vi "HEWH Assemble HEWH Diagnostics Data.vi"(8 "Error In":errorcluster, 11 "Water Heater GEA2 Data in":T1 {"Hyperterminal Data"."CRC" format="%x"; "Hyperterminal Data"."Length" format="%x"; "Hyperterminal Data"."Command" format="%x"; "Hyperterminal Data"."Destination" format="%x"; "Hyperterminal Data"."Source" format="%x"}) -> (0 "Error Out":errorcluster, 3 "Hyperterminal Data":string[][](array[string]))   [LabVIEW 2018]
uses:
  Utility/GEA2 Commands/HEWH/Type Definitions/GEA2 Commands WaterHeater GEA2 Data.ctl
  Utility/GEA2 Commands/HEWH/Type Definitions/GEA2 Commands Button Status.ctl
  Utility/GEA2 Commands/HEWH/Type Definitions/GEA2 Commands Status Query.ctl
  Utility/GEA2 Commands/HEWH/Type Definitions/GEA2 Commands Service Error Codes.ctl
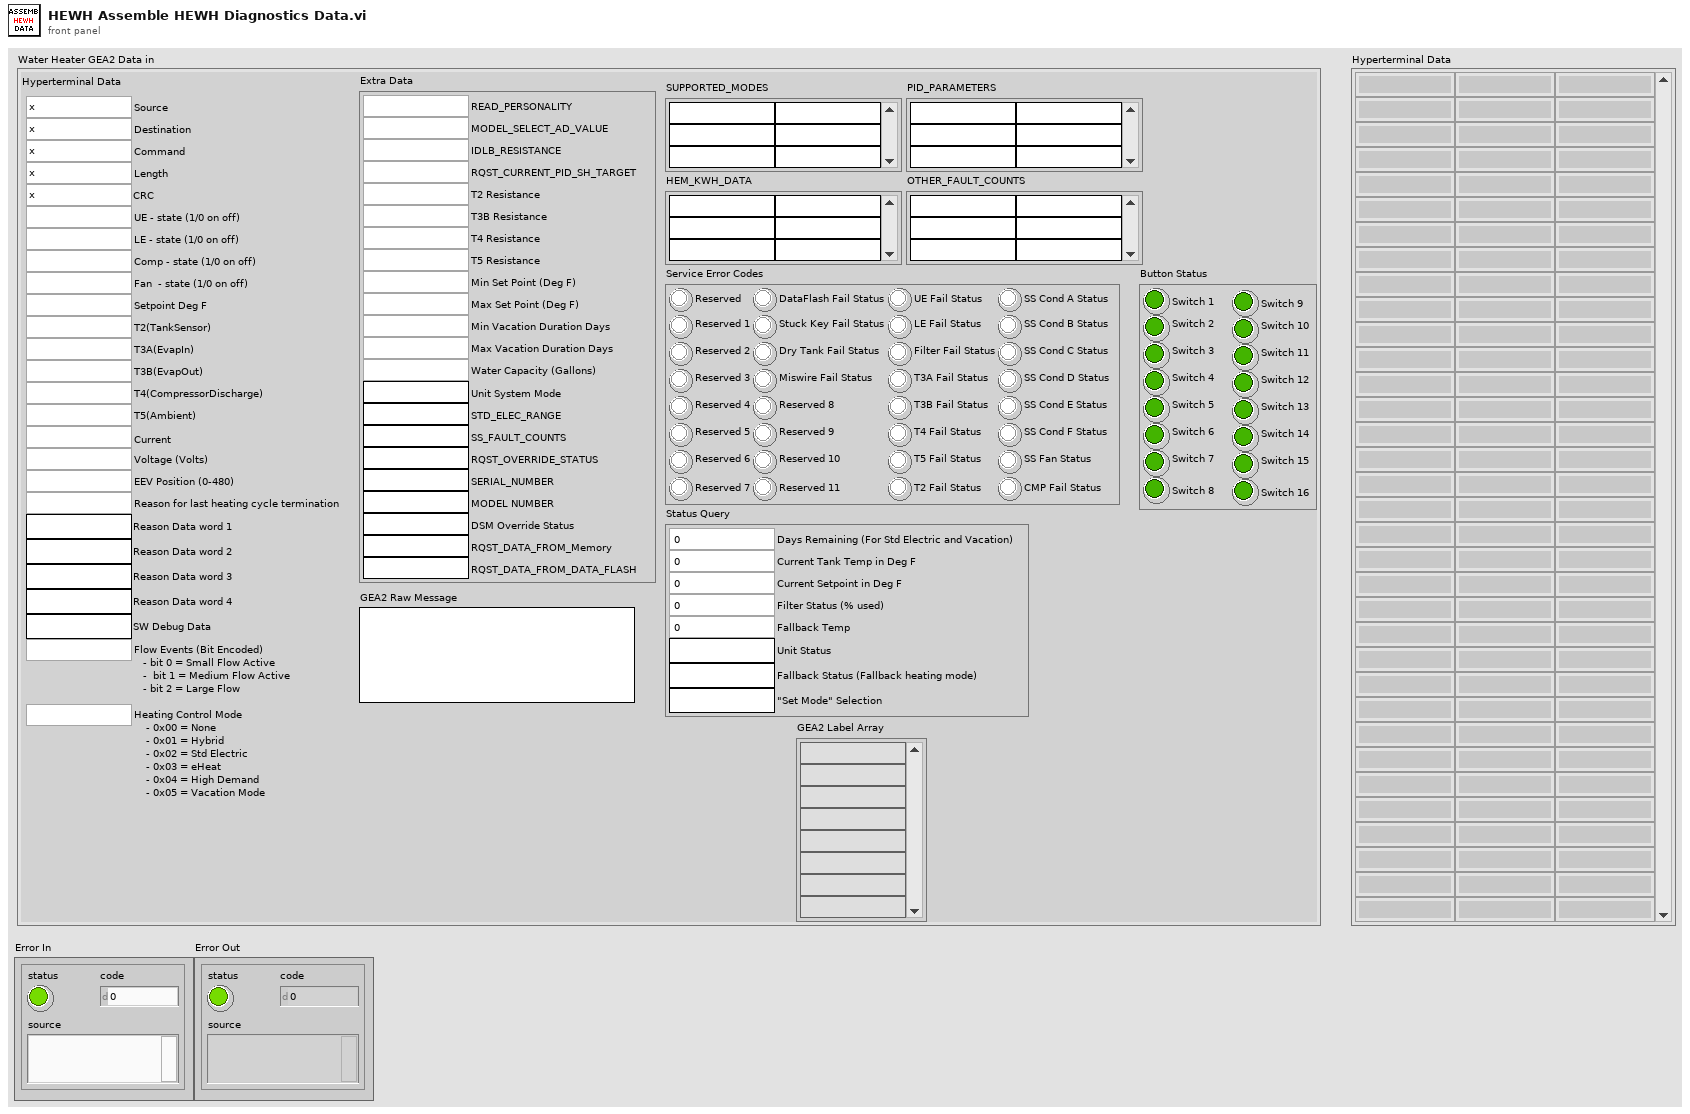
[diagram p1: front panel]
types:
  T1 = typedef "GEA2 Commands WaterHeater GEA2 Data.ctl" = cluster{"GEA2 Label Array":string[], "PID_PARAMETERS":string[][], "SUPPORTED_MODES":string[][], "Button Status":T2, "Status Query":T3, "Service Error Codes":T4, "HEM_KWH_DATA":string[][], "OTHER_FAULT_COUNTS":string[][], "GEA2 Raw Message":string, "Hyperterminal Data":cluster{"Source":u8, "Destination":u8, "Command":u8, "Length":u8, "CRC":u16, "UE - state (1/0 on off)":u8, "LE - state (1/0 on off)":u8, "Comp - state (1/0 on off)":u8, "Fan  - state (1/0 on off)":u8, "Setpoint Deg F":i32, "T2(TankSensor)":dbl, "T3A(EvapIn)":dbl, "T3B(EvapOut)":dbl, "T4(CompressorDischarge)":dbl, "T5(Ambient)":dbl, "Current":dbl, "Voltage (Volts)":u16, "EEV Position (0-480)":u16, "Reason for last heating cycle termination":u16, "Reason Data word 1":string, "Reason Data word 2":string, "Reason Data word 3":string, "Reason Data word 4":string, "SW Debug Data":string, "Flow Events (Bit Encoded)":u16, "Heating Control Mode":u16}, "Extra Data":cluster{"Water Capacity (Gallons)":u32, "Max Vacation Duration Days":u32, "Min Vacation Duration Days":u32, "Max Set Point (Deg F)":u32, "Min Set Point (Deg F)":u32, "T5 Resistance":u32, "T4 Resistance":u32, "T3B Resistance":u32, "T2 Resistance":u32, "STD_ELEC_RANGE":string, "SS_FAULT_COUNTS":string, "SERIAL_NUMBER":string, "READ_PERSONALITY":u8, "RQST_OVERRIDE_STATUS":string, "MODEL_SELECT_AD_VALUE":u32, "MODEL NUMBER":string, "IDLB_RESISTANCE":u32, "DSM Override Status":string, "RQST_DATA_FROM_Memory":string, "RQST_DATA_FROM_DATA_FLASH":string, "RQST_CURRENT_PID_SH_TARGET":u16, "Unit System Mode":string}}
  T2 = typedef "GEA2 Commands Button Status.ctl" = cluster{"Switch 1":bool, "Switch 2":bool, "Switch 3":bool, "Switch 4":bool, "Switch 5":bool, "Switch 6":bool, "Switch 7":bool, "Switch 8":bool, "Switch 9":bool, "Switch 10":bool, "Switch 11":bool, "Switch 12":bool, "Switch 13":bool, "Switch 14":bool, "Switch 15":bool, "Switch 16":bool}
  T3 = typedef "GEA2 Commands Status Query.ctl" = cluster{"Days Remaining (For Std Electric and Vacation)":u8, "Unit Status":string, "Current Tank Temp in Deg F":u8, "Current Setpoint in Deg F":u8, "Filter Status (% used)":u8, "Fallback Status (Fallback heating mode)":string, "Fallback Temp":u8, "\"Set Mode\" Selection":string}
  T4 = typedef "GEA2 Commands Service Error Codes.ctl" = cluster{"Reserved":bool, "Reserved 1":bool, "Reserved 2":bool, "Reserved 3":bool, "Reserved 4":bool, "Reserved 5":bool, "Reserved 6":bool, "Reserved 7":bool, "DataFlash Fail Status":bool, "Stuck Key Fail Status":bool, "Dry Tank Fail Status":bool, "Miswire Fail Status":bool, "Reserved 8":bool, "Reserved 9":bool, "Reserved 10":bool, "Reserved 11":bool, "UE Fail Status":bool, "LE Fail Status":bool, "Filter Fail Status":bool, "T3A Fail Status":bool, "T3B Fail Status":bool, "T4 Fail Status":bool, "T5 Fail Status":bool, "T2 Fail Status":bool, "SS Cond A Status":bool, "SS Cond B Status":bool, "SS Cond C Status":bool, "SS Cond D Status":bool, "SS Cond E Status":bool, "SS Cond F Status":bool, "SS Fan Status":bool, "CMP Fail Status":bool}
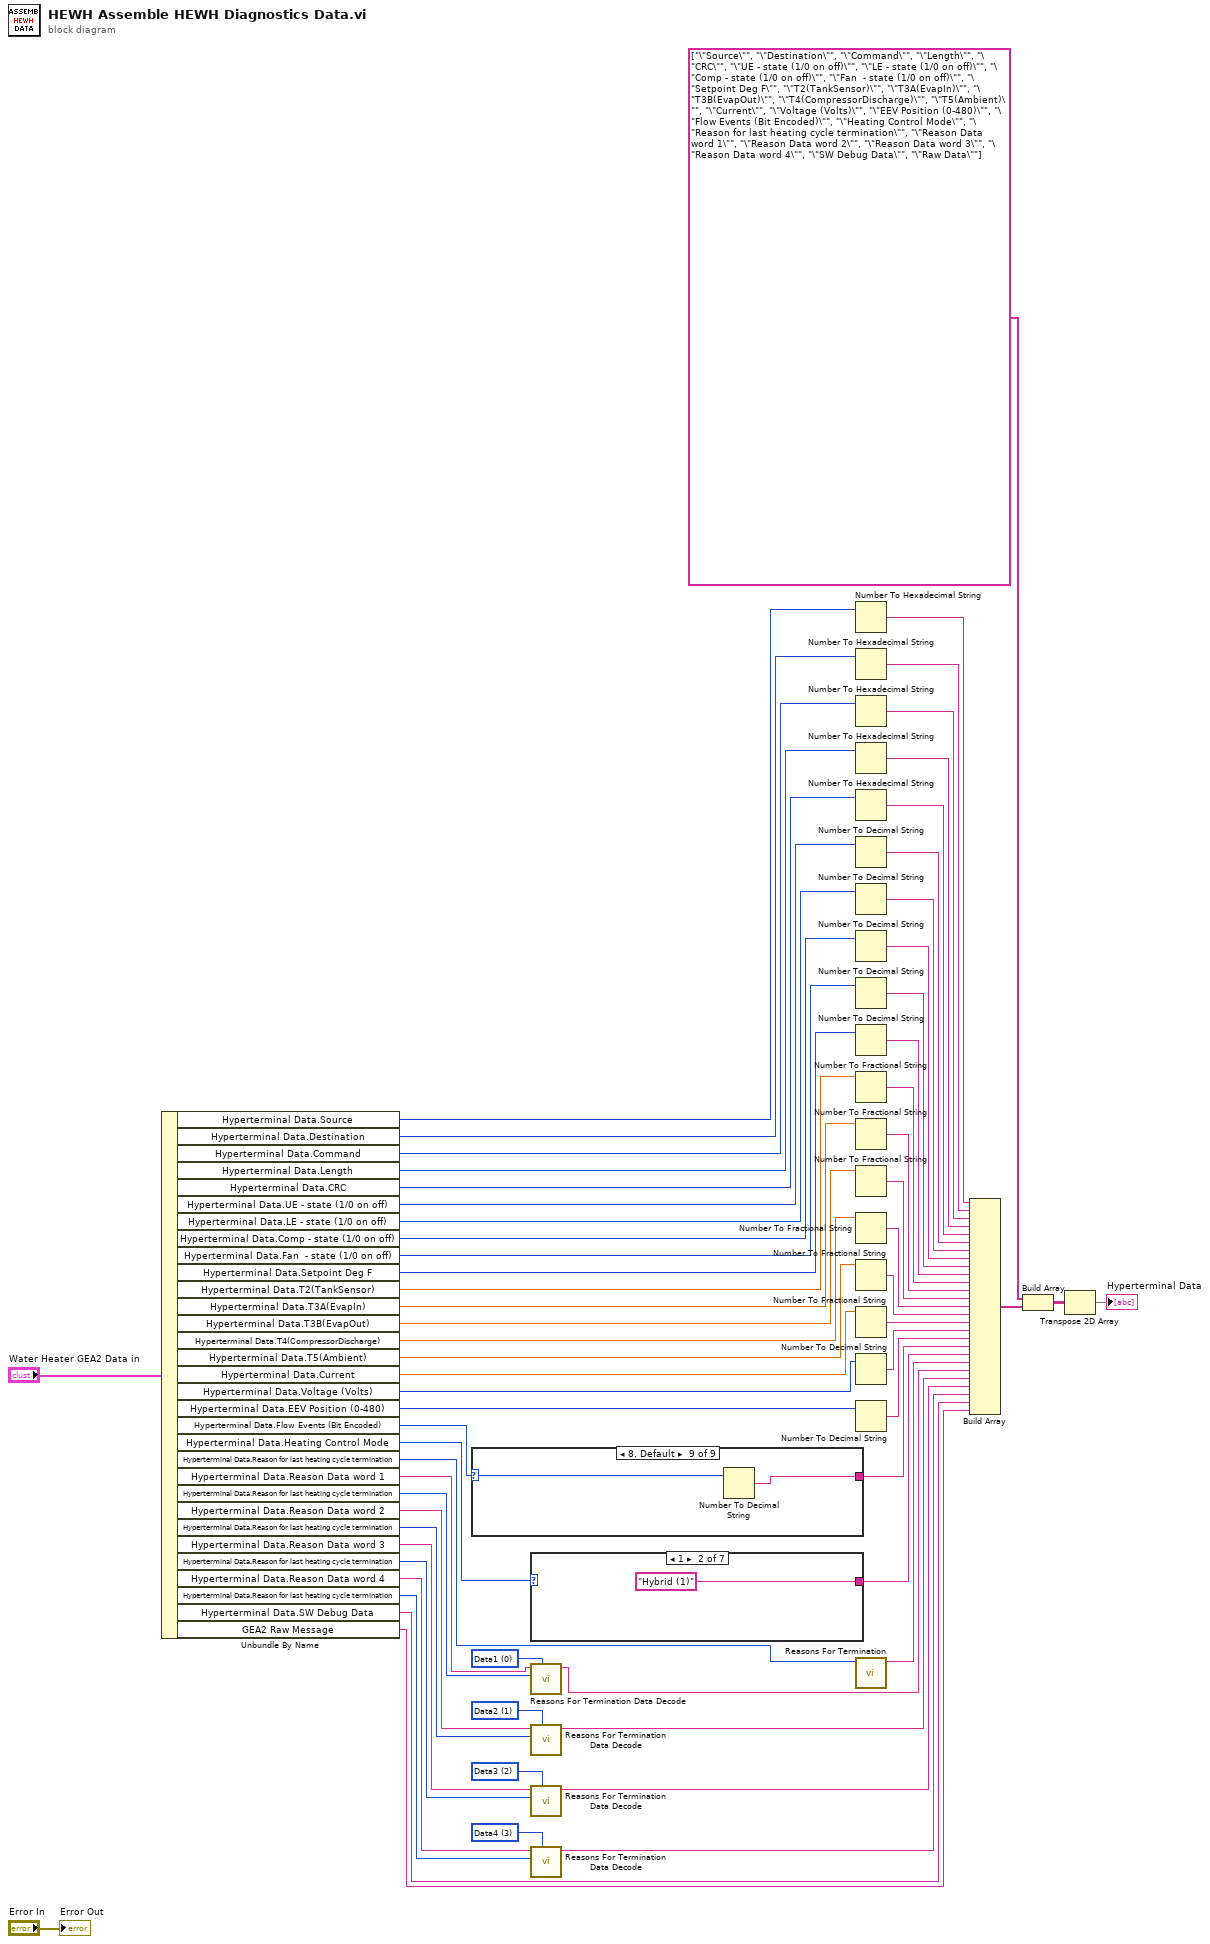
[diagram p0: block diagram]
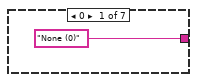
[diagram p2: hidden frame]
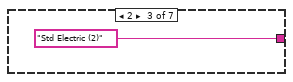
[diagram p3: hidden frame]
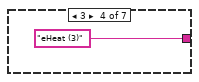
[diagram p4: hidden frame]
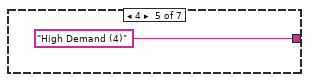
[diagram p5: hidden frame]
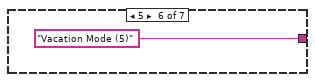
[diagram p6: hidden frame]
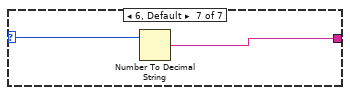
[diagram p7: hidden frame]
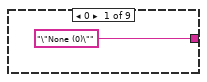
[diagram p8: hidden frame]
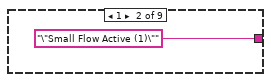
[diagram p9: hidden frame]
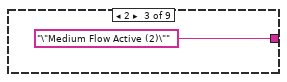
[diagram p10: hidden frame]
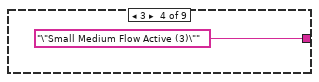
[diagram p11: hidden frame]
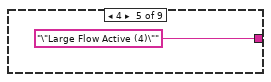
[diagram p12: hidden frame]
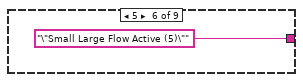
[diagram p13: hidden frame]
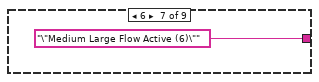
[diagram p14: hidden frame]
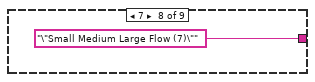
[diagram p15: hidden frame]
diagram:
  w23 = u16 3 items=["Data1", "Data2", "Data3", "Data4"] ("Data")
  w22 = u16 2 items=["Data1", "Data2", "Data3", "Data4"] ("Data")
  w21 = u16 1 items=["Data1", "Data2", "Data3", "Data4"] ("Data")
  w20 = u16 0 items=["Data1", "Data2", "Data3", "Data4"] ("Data")
  n1 = Unbundle By Name("Water Heater GEA2 Data in") -> ("Hyperterminal Data.Source"=w2:u8, "Hyperterminal Data.Destination"=w3:u8, "Hyperterminal Data.Command"=w4:u8, "Hyperterminal Data.Length"=w5:u8, "Hyperterminal Data.CRC"=w6:u16, "Hyperterminal Data.UE - state (1/0 on off)"=w7:u8, "Hyperterminal Data.LE - state (1/0 on off)"=w8:u8, "Hyperterminal Data.Comp - state (1/0 on off)"=w9:u8, "Hyperterminal Data.Fan  - state (1/0 on off)"=w10:u8, "Hyperterminal Data.Setpoint Deg F"=w11:i32, "Hyperterminal Data.T2(TankSensor)"=w12:dbl, "Hyperterminal Data.T3A(EvapIn)"=w13:dbl, "Hyperterminal Data.T3B(EvapOut)"=w14:dbl, "Hyperterminal Data.T4(CompressorDischarge)"=w15:dbl, "Hyperterminal Data.T5(Ambient)"=w16:dbl, "Hyperterminal Data.Current"=w17:dbl, "Hyperterminal Data.Voltage (Volts)"=w18:u16, "Hyperterminal Data.EEV Position (0-480)"=w19:u16, "Hyperterminal Data.Flow Events (Bit Encoded)"=w48:u16, "Hyperterminal Data.Heating Control Mode"=w61:u16, "Hyperterminal Data.Reason for last heating cycle termination"=w54:u16, "Hyperterminal Data.Reason Data word 1"=w63:string, "Hyperterminal Data.Reason for last heating cycle termination"=w55:u16, "Hyperterminal Data.Reason Data word 2"=w64:string, "Hyperterminal Data.Reason for last heating cycle termination"=w56:u16, "Hyperterminal Data.Reason Data word 3"=w65:string, "Hyperterminal Data.Reason for last heating cycle termination"=w57:u16, "Hyperterminal Data.Reason Data word 4"=w66:string, "Hyperterminal Data.Reason for last heating cycle termination"=w58:u16, "Hyperterminal Data.SW Debug Data"=w47:string, "GEA2 Raw Message"=w49:string)
  n2 = case shown="8, Default" w48 {
    selector: w48 -> [_ _ _ _ _ _ _ _ w76]
    tunnel: ["\"None (0)\"" "\"Small Flow Active (1)\"" "\"Medium Flow Active (2)\"" "\"Small Medium Flow Active (3)\"" "\"Large Flow Active (4)\"" "\"Small Large Flow Active (5)\"" "\"Medium Large Flow Active (6)\"" "\"Small Medium Large Flow (7)\"" w75] -> w60
    frame 0 {
    }
    frame 1 {
    }
    frame 2 {
    }
    frame 3 {
    }
    frame 4 {
    }
    frame 5 {
    }
    frame 6 {
    }
    frame 7 {
    }
    frame 8, Default {
      n3 = Number To Decimal String(number=w76) -> (decimal integer string=w75:string)  [unwired: 1 in]
    }
  }
  n4 = case shown="1" w61 {
    selector: w61 -> [_ _ _ _ _ _ w84]
    tunnel: ["None (0)" "Hybrid (1)" "Std Electric (2)" "eHeat (3)" "High Demand (4)" "Vacation Mode (5)" w83] -> w62
    frame 0 {
    }
    frame 1 {
    }
    frame 2 {
    }
    frame 3 {
    }
    frame 4 {
    }
    frame 5 {
    }
    frame 6, Default {
      n5 = Number To Decimal String(number=w84) -> (decimal integer string=w83:string)  [unwired: 1 in]
    }
  }
  n6 = call "Reasons For Termination Data Decode.vi"("Data"=w20, "Reason for Last Heating Cycle Termination"=w55, "Reason Data Word"=w63) -> ("Reason Data Word 1 Output"=w43:string)  [unwired: 8 in]
  n7 = call "Reasons For Termination Data Decode.vi"("Data"=w21, "Reason for Last Heating Cycle Termination"=w56, "Reason Data Word"=w64) -> ("Reason Data Word 1 Output"=w44:string)  [unwired: 8 in]
  n8 = call "Reasons For Termination Data Decode.vi"("Data"=w22, "Reason for Last Heating Cycle Termination"=w57, "Reason Data Word"=w65) -> ("Reason Data Word 1 Output"=w45:string)  [unwired: 8 in]
  n9 = call "Reasons For Termination Data Decode.vi"("Data"=w23, "Reason for Last Heating Cycle Termination"=w58, "Reason Data Word"=w66) -> ("Reason Data Word 1 Output"=w46:string)  [unwired: 8 in]
  n10 = Number To Hexadecimal String(2:w2) -> (0:w24:string)  [unwired: 1 in]
  n11 = Number To Hexadecimal String(2:w3) -> (0:w25:string)  [unwired: 1 in]
  n12 = Number To Hexadecimal String(2:w4) -> (0:w26:string)  [unwired: 1 in]
  n13 = Number To Hexadecimal String(2:w5) -> (0:w27:string)  [unwired: 1 in]
  n14 = Number To Hexadecimal String(2:w6) -> (0:w28:string)  [unwired: 1 in]
  n15 = Number To Decimal String(number=w7) -> (decimal integer string=w29:string)  [unwired: 1 in]
  n16 = Number To Decimal String(number=w8) -> (decimal integer string=w30:string)  [unwired: 1 in]
  n17 = Number To Decimal String(number=w9) -> (decimal integer string=w31:string)  [unwired: 1 in]
  n18 = Number To Decimal String(number=w10) -> (decimal integer string=w32:string)  [unwired: 1 in]
  n19 = Number To Decimal String(number=w11) -> (decimal integer string=w33:string)  [unwired: 1 in]
  n20 = Number To Fractional String(number=w12) -> (F-format string=w34:string)  [unwired: 3 in]
  n21 = Number To Fractional String(number=w13) -> (F-format string=w35:string)  [unwired: 3 in]
  n22 = Number To Fractional String(number=w14) -> (F-format string=w36:string)  [unwired: 3 in]
  n23 = Number To Fractional String(number=w15) -> (F-format string=w37:string)  [unwired: 3 in]
  n24 = Number To Fractional String(number=w16) -> (F-format string=w38:string)  [unwired: 3 in]
  n25 = Number To Fractional String(number=w17) -> (F-format string=w39:string)  [unwired: 3 in]
  n26 = Number To Decimal String(number=w18) -> (decimal integer string=w40:string)  [unwired: 1 in]
  n27 = Number To Decimal String(number=w19) -> (decimal integer string=w41:string)  [unwired: 1 in]
  n28 = call "Reasons For Termination.vi"("Reason for last heating cycle termination"=w54) -> ("String"=w42:string)  [unwired: 10 in]
  n29 = Build Array(w24, w25, w26, w27, w28, w29, w30, w31, w32, w33, w34, w35, w36, w37, w38, w39, w40, w41, w60, w62, w42, w43, w44, w45, w46, w47, w49) -> (w50:string[])
  n30 = Build Array(string[] ["\"Source\"", "\"Destination\"", "\"Command\"", "\"Length\"", "\"CRC\"", "\"UE - state (1/0 on off)\"", "\"LE - state (1/0 on off)\"", "\"Comp - state (1/0 on off)\"", "\"Fan  - state (1/0 on off)\"", "\"Setpoint Deg F\"", "\"T2(TankSensor)\"", "\"T3A(EvapIn)\"", "\"T3B(EvapOut)\"", "\"T4(CompressorDischarge)\"", "\"T5(Ambient)\"", "\"Current\"", "\"Voltage (Volts)\"", "\"EEV Position (0-480)\"", "\"Flow Events (Bit Encoded)\"", "\"Heating Control Mode\"", "\"Reason for last heating cycle termination\"", "\"Reason Data word 1\"", "\"Reason Data word 2\"", "\"Reason Data word 3\"", "\"Reason Data word 4\"", "\"SW Debug Data\"", "\"Raw Data\""] ("GEA2 Label Array"), w50) -> (w52:string[][])
  n31 = Transpose 2D Array(2D array=w52) -> (transposed array=→"Hyperterminal Data":string[][])
  "Error Out" <- "Error In"
